vi "acc_est.vi"() -> ()   [LabVIEW 2021]
uses:
  <vilib>/myRIO/Instrument Drivers/Onboard IO/I2C/typedefs/I2C User Configuration.ctl
  <vilib>/myRIO/Instrument Drivers/Onboard IO/I2C/typedefs/I2C Transfer Rate.ctl
  <vilib>/Platform/TimedLoop/XDataNode/timing_clust.ctl
  <vilib>/Platform/TimedLoop/XDataNode/nitl_modes.ctl
  <vilib>/Platform/TimedLoop/XDataNode/wakeup.ctl
  <vilib>/myRIO/Instrument Drivers/Onboard IO/DIO/typedefs/DIO Reference.ctl
  <vilib>/myRIO/Common/Instrument Driver Framework/Utilities/typedefs/myRIO Generic Hardware Reference.ctl
  <vilib>/myRIO/Common/Instrument Driver Framework/Utilities/typedefs/Hardware Version Enum.ctl
  <vilib>/myRIO/Common/Instrument Driver Framework/Utilities/typedefs/myRIO v1.0 Reference.ctl
  <vilib>/myRIO/Common/Instrument Driver Framework/Utilities/typedefs/Generic FPGA Reference.ctl
  <vilib>/myRIO/Common/Instrument Driver Framework/myRIO v1.0/DIO/typedefs/DIO Channels List.ctl
  <vilib>/myRIO/Common/Instrument Driver Framework/myRIO v1.0/DIO/typedefs/DIO Channels Enum.ctl
  <vilib>/userDefined/High Color/nirio_resource_hc.ctl
  <vilib>/myRIO/Instrument Drivers/Onboard IO/I2C/typedefs/I2C Reference.ctl
  <vilib>/myRIO/Common/Instrument Driver Framework/myRIO v1.0/I2C/typedefs/I2C Channels Enum.ctl
  <vilib>/myRIO/Instrument Drivers/Onboard IO/I2C/typedefs/I2C Configuration.ctl
  <vilib>/myRIO/Common/Instrument Driver Framework/myRIO v1.0/DIO/vis/myRIO v1.1 Open DIO.vi
  <vilib>/myRIO/Common/Instrument Driver Framework/myRIO v1.0/I2C/vis/myRIO v1.1 Open I2C.vi
  <vilib>/myRIO/Common/Instrument Driver Framework/Utilities/vis/Validate Channels.vi
  <vilib>/myRIO/Common/Instrument Driver Framework/myRIO v1.0/DIO/vis/myRIO v1.0 Reserve DIO.vi
  <vilib>/myRIO/Common/Instrument Driver Framework/myRIO v1.0/I2C/vis/myRIO v1.0 Reserve I2C.vi
  <vilib>/myRIO/Common/Instrument Driver Framework/myRIO v1.0/UART/vis/myRIO v1.0 Close UART.vi
  <vilib>/myRIO/Common/Instrument Driver Framework/myRIO v1.0/Resource Manager/vis/myRIO v1.0 Reserve Channel List.vi
  <vilib>/myRIO/Common/Instrument Driver Framework/myRIO v1.0/DIO/vis/myRIO v1.0 Build MUX Configuration DIO.vi
  <vilib>/myRIO/Common/Instrument Driver Framework/myRIO v1.0/I2C/vis/myRIO v1.0 Build MUX Configuration I2C.vi
  <vilib>/myRIO/Common/Instrument Driver Framework/myRIO v1.0/Resource Manager/vis/myRIO v1.0 Reserve Channel.vi
  <vilib>/myRIO/Common/Instrument Driver Framework/myRIO v1.0/Resource Manager/vis/myRIO v1.0 Unreserve Channel.vi
  <vilib>/myRIO/Common/Instrument Driver Framework/myRIO v1.0/Resource Manager/vis/myRIO v1.0 Create Configuration List.vi
  <vilib>/myRIO/Common/Instrument Driver Framework/myRIO v1.0/Resource Manager/vis/myRIO v1.0 Build Mutex Name.vi
  <vilib>/Utility/VariantDataType/GetNumericInfo.vi
  <vilib>/Utility/error.llb/Error Cluster From Error Code.vi
  <vilib>/myRIO/Common/Instrument Driver Framework/myRIO v1.0/myRIO v1.1 Open.vi
  <vilib>/myRIO/Common/Instrument Driver Framework/Utilities/vis/IO Manager.vi
  <vilib>/myRIO/Common/Instrument Driver Framework/Utilities/vis/Configuration Manager.vi
  <vilib>/myRIO/Common/Instrument Driver Framework/myRIO v1.0/Resource Manager/vis/myRIO v1.0 Configure IO.vi
  <vilib>/myRIO/Common/Instrument Driver Framework/myRIO v1.0/myRIO v1.0 Close.vi
  <vilib>/myRIO/Common/Instrument Driver Framework/myRIO v1.0/I2C/vis/myRIO v1.0 Configure I2C.vi
  <vilib>/myRIO/Common/Instrument Driver Framework/myRIO v1.0/I2C/vis/myRIO v1.0 Write I2C.vi
  <vilib>/myRIO/Common/Instrument Driver Framework/myRIO v1.0/DIO/vis/myRIO v1.0 Read DIO.vi
  <vilib>/myRIO/Common/Instrument Driver Framework/myRIO v1.0/I2C/vis/myRIO v1.0 Read I2C.vi
  <vilib>/myRIO/Common/Instrument Driver Framework/myRIO v1.0/DIO/vis/myRIO v1.0 Write DIO.vi
  <vilib>/myRIO/Common/Instrument Driver Framework/Utilities/vis/FPGA Ref Manager.vi
  <vilib>/myRIO/Common/Instrument Driver Framework/myRIO v1.0/myRIO v1.0 Reset FPGA.vi
  <vilib>/myRIO/Common/Instrument Driver Framework/myRIO v1.0/IRQ/vis/myRIO v1.0 IRQ Info FGV.vi
  <vilib>/myRIO/Common/Instrument Driver Framework/myRIO v1.0/IRQ/vis/myRIO v1.0 Timer IRQ Info FGV.vi
  <vilib>/myRIO/Common/Instrument Driver Framework/myRIO v1.0/IRQ/vis/myRIO v1.0 ISR Agent.vi
  <vilib>/myRIO/Instrument Drivers/Utilities/vis/Reset Index.vi
  <vilib>/myRIO/Common/Instrument Driver Framework/myRIO v1.0/Resource Manager/vis/myRIO v1.0 Block Write Resource Manager.vi
  <vilib>/myRIO/Instrument Drivers/Onboard IO/I2C/vis/myRIO I2C Open.xnode
  <vilib>/myRIO/Instrument Drivers/Onboard IO/DIO/vis/myRIO DIO Open.xnode
  <vilib>/platform/TimedLoop/XDataNode/XDataNode.xnode
  <vilib>/myRIO/Instrument Drivers/Onboard IO/I2C/I2C.lvlib
  <vilib>/myRIO/Instrument Drivers/Onboard IO/DIO/DIO.lvlib
  <vilib>/Platform/TimedLoop/XDataNode/XDNodeRunTimeDep.lvlib
  <vilib>/myRIO/Instrument Drivers/Utilities/Utilities.lvlib
panel:
  in  "stop":bool
  out "INT_Source":bool[](array[boolean])
  out "Waveform Chart":cluster{i16, i16, i16}(graph)
  out "Z":i16
  out "Y":i16
  out "X":i16
  out "Bytes Read":u8[](array[numeric]) format="%x"
  # "2T"
  # "A"
  # "I"
  # "D"
  # "1T"
  # "O"
  # "F"
  # "W"
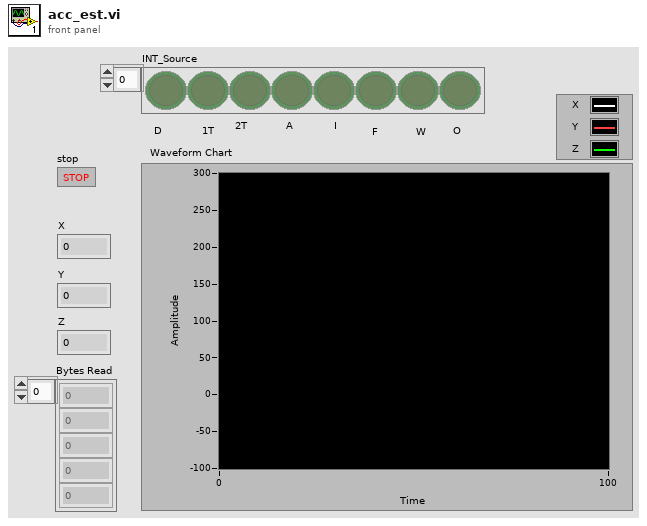
[diagram p1: front panel]
types:
  T1 = typedef "I2C.lvlib/I2C User Configuration.ctl" = cluster{"I2C Transfer Rate":T2}
  T2 = typedef "I2C.lvlib/I2C Transfer Rate.ctl" = enum16{"Standard mode (100 kbps)", "Fast mode (400 kbps)"}
  T3 = typedef "I2C.lvlib/I2C Reference.ctl" = cluster{"myRIO Reference":T4, "I2C Channels Enum":T8, "I2C Configuration":T9}
  T4 = typedef "myRIO Generic Hardware Reference.ctl" = cluster{"myRIO Model":T5, "myRIO Hardware Reference":T6}
  T5 = typedef "Hardware Version Enum.ctl" = enum16{"Unknown", "myRIO-1900", "myRIO-1950", "roboRIO", "NI ELVIS RIO CM", "ELVIS III"}
  T6 = typedef "myRIO v1.0 Reference.ctl" = cluster{"Generic FPGA Reference":T7, "Allow multiple opens":bool}
  T7 = typedef "Generic FPGA Reference.ctl" = refnum<k20>
  T8 = typedef "I2C Channels Enum.ctl" = enum16{"Not Connected", "A/I2C", "B/I2C", "I2C/I2C"}
  T9 = typedef "I2C.lvlib/I2C Configuration.ctl" = cluster{"I2C Transfer Rate":T2}
  T10 = typedef "DIO.lvlib/DIO Reference.ctl" = cluster{"myRIO Reference":T4, "DIO Channels List":T11}
  T11 = typedef "DIO Channels List.ctl" = T12[]
  T12 = typedef "DIO Channels Enum.ctl" = enum16{"Not Connected", "C/DIO0", "C/DIO1", "C/DIO2", "C/DIO3", "C/DIO4", "C/DIO5", "C/DIO6", "C/DIO7", "A/DIO0", "A/DIO1", "A/DIO2", "A/DIO3", "A/DIO4", "A/DIO5", "A/DIO6", "A/DIO7", "A/DIO8", "A/DIO9", "A/DIO10", "A/DIO11", "A/DIO12", "A/DIO13", "A/DIO14", "A/DIO15", "A/DIO16", "A/DIO17", "A/DIO18", "A/DIO19", "B/DIO0", "B/DIO1", "B/DIO2", "B/DIO3", "B/DIO4", "B/DIO5", "B/DIO6", "B/DIO7", "B/DIO8", "B/DIO9", "B/DIO10", "B/DIO11", "B/DIO12", "B/DIO13", "B/DIO14", "B/DIO15", "B/DIO16", "B/DIO17", "B/DIO18", "B/DIO19", "LED0", "LED1", "LED2", "LED3", "Button0", "DIO/DIO0", "DIO/DIO1", "DIO/DIO2", "DIO/DIO3", "DIO/DIO4", "DIO/DIO5", "DIO/DIO6", "DIO/DIO7", "DIO/DIO8", "DIO/DIO9", "SPI/CS0", "SPI/CS1", "SPI/CS2", "SPI/CS3", "LED RADIO (Green)", "LED RADIO (Red)", "LED COMM (Green)", "LED COMM (Red)", "LED MODE (Green)", "LED MODE (Red)"}
  T13 = typedef "XDNodeRunTimeDep.lvlib/timing_clust.ctl" = cluster{"Expected End [f-1]":u64, "Actual End [f-1]":u64, "Finished Late? [f-1]":bool, "Expected End [i-1]":u64, "Actual End [i-1]":u64, "Finished Late? [i-1]":bool, "Expected Start [i]":u64, "Actual Start [i]":u64, "Expected Start [f]":u64, "Actual Start [f]":u64, "Source Name":string, "Structure Name":string, "Period":i64, "Deadline":i64, "Offset":i64, "Start":i64, "Priority":i32, "Timeout":i32, "Mode":T14, "Wakeup Reason":T15, "Error":errorcluster, "Source Type":string, "Secondary Source Type":string, "Global End Time":u64, "Global Start Time":u64, "Frame Duration":u64, "Iteration Duration":u64, "Assigned CPU":i32, "I/O Scan Engine Mode":u32}
  T14 = typedef "XDNodeRunTimeDep.lvlib/nitl_modes.ctl" = enum32{"No Change", "Process missed periods, maintain original phase", "Discard missed periods, maintain original phase", "Process missed periods, ignore original phase", "Discard missed periods, ignore original phase"}
  T15 = typedef "XDNodeRunTimeDep.lvlib/wakeup.ctl" = enum32{"Normal", "Aborted", "Asynchronous wakeup", "Timing source error", "Timed loop error", "Timeout"}
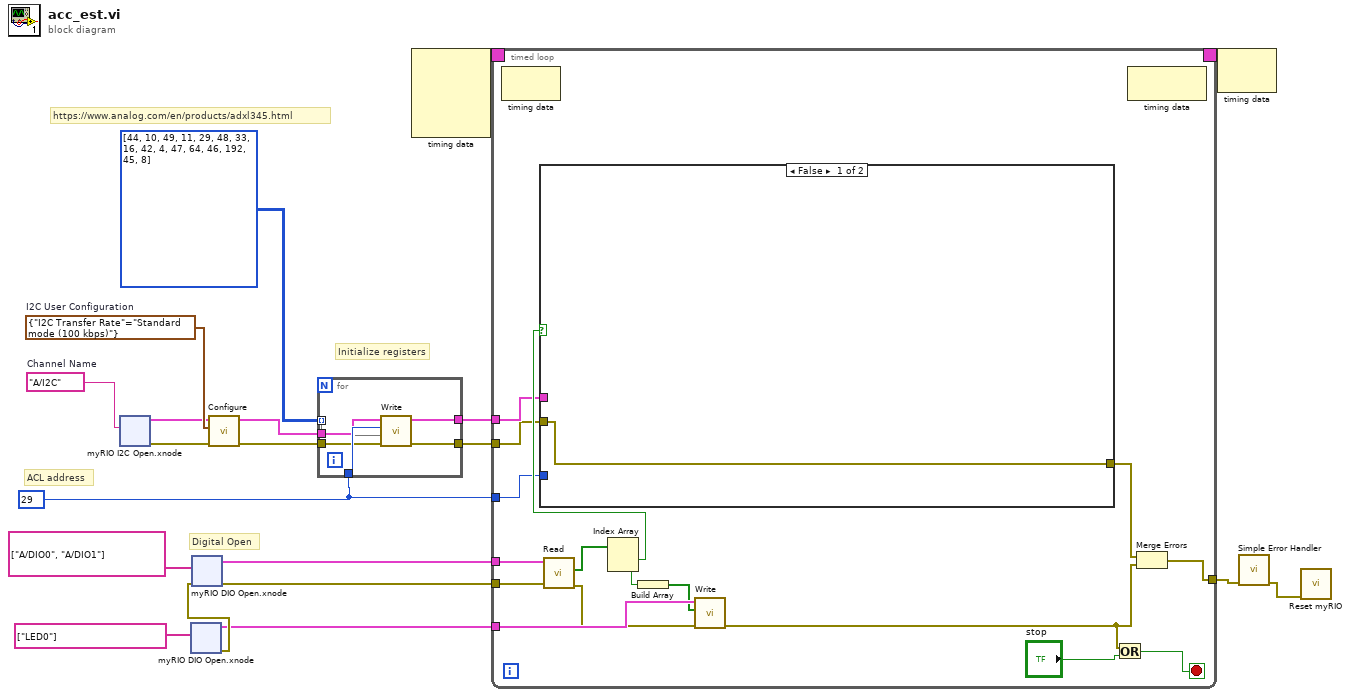
[diagram p0: block diagram]
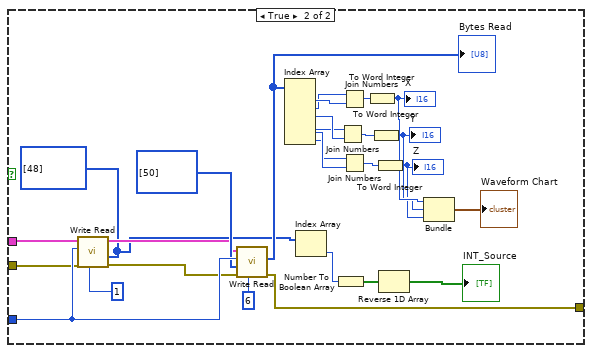
[diagram p2: hidden frame]
diagram:
  w4 = u8 29 ("Slave Address (7-bit)")
  w19 = T1 {"I2C Transfer Rate"=enum."Standard mode (100 kbps)"}  # I2C User Configuration
  w20 = tag "A/I2C"  # Channel Name
  # "Digital Open"
  # "ACL address"
  # "https://www.analog.com/en/products/adxl345.html"
  # "Initialize registers"
  n1 = xnode "myRIO I2C Open.xnode"("Channel Name"=w20) -> ("error out"=w17:errorcluster, "I2C Ref Out"=w18:T3)  [unwired: 2 in]
  n2 = xnode "myRIO DIO Open.xnode"("Channel Names"=tag[] ["LED0"]) -> ("error out"=w11:errorcluster, "DIO Ref Out"=w9:T10)  [unwired: 2 in]
  n3 = xnode "myRIO DIO Open.xnode"("error in (no error)"=w11, "Channel Names"=tag[] ["A/DIO0", "A/DIO1"]) -> ("error out"=w8:errorcluster, "DIO Ref Out"=w10:T10)  [unwired: 1 in]
  n4 = call <vilib>:"Configure.vi"("error in (no error)"=w17, "I2C User Configuration"=w19, "I2C Ref In"=w18) -> ("error out"=w15:errorcluster, "I2C Ref Out"=w16:T3)  [unwired: 7 in]
  n5 = for {
    tunnel: w4 -> [w26]
    tunnel: w16 -> [w25]
    tunnel: w15 -> [w24]
    tunnel: i32[][] [[44, 10], [49, 11], [29, 48], [33, 16], [42, 4], [47, 64], [46, 192], [45, 8]] -> [w23] mode=indexing
    tunnel: [w22] -> w5
    tunnel: [w21] -> w3
    n6 = call <vilib>:"Write.vi"("error in (no error)"=w24, "Bytes to Write"=w23, "Slave Address (7-bit)"=w26, "I2C Ref In"=w25) -> ("error out"=w21:errorcluster, "I2C Ref Out"=w22:T3)  [unwired: 6 in]
  }
  n7 = node-c288() -> (w7:T13)  [unwired: 4 in]
  n8 = timed-loop {
    tunnel: w10 -> [w42]
    tunnel: w9 -> [w41]
    tunnel: w8 -> [w40]
    timing: w7 -> [_]
    timing-out: [_] -> w6
    tunnel: w5 -> [w34]
    tunnel: w4 -> [w33]
    tunnel: w3 -> [w32]
    tunnel: [w30] -> w2
    stop <- w29 stop-if-true
    n9 = node-c288() -> ()  [unwired: 1 in, 1 out]
    n10 = call <vilib>:"Read.vi"("error in (no error)"=w40, "DIO Ref In"=w42) -> ("error out"=w39:errorcluster, "Values"=w38:bool[])  [unwired: 7 in, 1 out]
    n11 = Index Array(array=w38) -> (element #1=w37:bool, element #2=w36:bool)  [unwired: 2 in]
    n12 = case shown="False" w37 {
      tunnel: w34 -> [_ w64]
      tunnel: w33 -> [_ w70]
      tunnel: w32 -> [w43 w45]
      tunnel: [w43 w44] -> w31
      frame False {
      }
      frame True {
        w49 = u8[] [48] ("Bytes to Write")
        n13 = call <vilib>:"Write Read.vi"("Byte Count"=u32 1, "error in (no error)"=w45, "Bytes to Write"=w49, "Slave Address (7-bit)"=w70, "I2C Ref In"=w64) -> ("error out"=w67:errorcluster, "I2C Ref Out"=w68:T3)  [unwired: 3 in, 1 out]
        n14 = call <vilib>:"Write Read.vi"("Byte Count"=u32 6, "error in (no error)"=w67, "Bytes to Write"=u8[] [50], "Slave Address (7-bit)"=w70, "I2C Ref In"=w68) -> ("error out"=w44:errorcluster, "Bytes Read"=w63:u8[])  [unwired: 3 in, 1 out]
        "Bytes Read" <- w63
        n15 = Index Array(array=w63) -> (element #1=w62:u8, element #2=w61:u8, element #3=w59:u8, element #4=w58:u8, element #5=w57:u8, element #6=w56:u8)  [unwired: 6 in]
        n16 = Index Array(array=w49) -> (element=w48:u8)  [unwired: 1 in]
        n17 = Number To Boolean Array(number=w48) -> (Boolean array=w47:bool[])
        n18 = Join Numbers(hi=w58, lo=w59) -> ((hi.lo)=w55:u16)
        n19 = Join Numbers(hi=w61, lo=w62) -> ((hi.lo)=w60:u16)
        n20 = Join Numbers(hi=w56, lo=w57) -> ((hi.lo)=w54:u16)
        n21 = To Word Integer(number=w60) -> (16bit integer=w53:i16)
        "X" <- w53
        n22 = To Word Integer(number=w55) -> (16bit integer=w52:i16)
        "Y" <- w52
        n23 = To Word Integer(number=w54) -> (16bit integer=w51:i16)
        "Z" <- w51
        n24 = Reverse 1D Array(array=w47) -> (reversed array=→"INT_Source":bool[])
        n25 = Bundle(w53, w52, w51) -> (→"Waveform Chart":cluster{i16, i16, i16})  [unwired: 1 in]
      }
    }
    n26 = Build Array(w36) -> (w35:bool[])
    n27 = call <vilib>:"Write.vi"("error in (no error)"=w39, "Values"=w35, "DIO Ref In"=w41) -> ("error out"=w27:errorcluster)  [unwired: 6 in, 1 out]
    n28 = Or(x=w27, y="stop") -> (x .or. y?=w29:bool)
    n29 = node-c288() -> ()  [unwired: 1 in, 1 out]
    n30 = Merge Errors(w31, w27) -> (w30:errorcluster)
  }
  n31 = node-c288(w6) -> ()  [unwired: 1 out]
  n32 = call <vilib>:"Simple Error Handler.vi"("error in (no error)"=w2) -> ("error out"=w1:errorcluster)  [unwired: 4 in, 4 out]
  n33 = call <vilib>:"Reset myRIO.vi"("error in (no error)"=w1) -> ()  [unwired: 10 in, 1 out]
